vi "Get Device ID.vi"(8 "Error In":errorcluster, 11 "LINX Device Config":T1) -> (0 "Error Out":errorcluster, 2 "Device Name":string, 3 "LINX Device Config":T1)   [LabVIEW 2011, in "LVH-LINX.lvlib" / "Device.lvlib"]
uses:
  Device.lvlib
  Type Defs/LINX Device Config.ctl
  Type Defs/Interface.ctl
  Type Defs/TCP Config.ctl
  Type Defs/Device Family.ctl
  Type Defs/Error Type.ctl
  LVH-LINX.lvlib
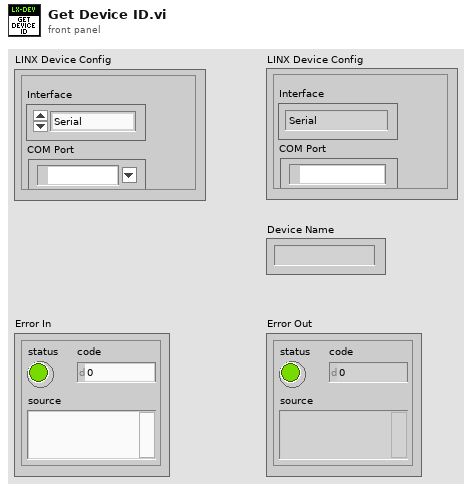
[diagram p1: front panel]
types:
  T1 = typedef "LVH-LINX.lvlib/Device.lvlib/LINX Device Config.ctl" = cluster{"Interface":T2, "COM Port":refnum<visa-resource-name>, "TCP Configuration":T3, "Device Family":T4, "Device ID":u8, "Device Name":string, "TCP Ref":refnum<k5>}
  T2 = typedef "LVH-LINX.lvlib/Interface.ctl" = enum16{"Serial", "TCP"}
  T3 = typedef "LVH-LINX.lvlib/Device.lvlib/TCP Config.ctl" = cluster{"IP Address":string, "Port":u16}
  T4 = typedef "LVH-LINX.lvlib/Device Family.ctl" = enum8{"National Instruments", "Digilent", "Arduino"}
  T5 = typedef "LVH-LINX.lvlib/Error Type.ctl" = enum16{"Unknown", "Timeout", "Corrupt Return Packet", "Unable To Connect", "Command Not Supported", "Channel DNE"}
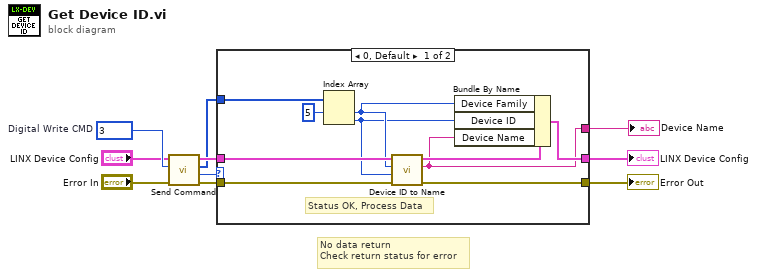
[diagram p0: block diagram]
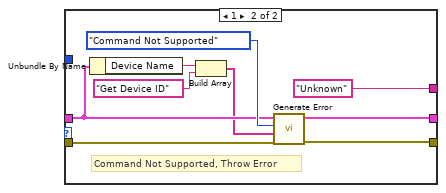
[diagram p2: hidden frame]
diagram:
  w9 = u16 3  # Digital Write CMD
  # "No data return\nCheck return status for error"
  n1 = call "Send Command.vi"("Error In"="Error In", "CMD"=w9, "LINX Device Config"="LINX Device Config") -> ("Error Out"=w4:errorcluster, "Status"=w1:u8, "Response"=w3:u8[], "LINX Device Config"=w6:T1)  [unwired: 5 in]
  n2 = case shown="0, Default" w1 {
    tunnel: [w14 w27] -> w7
    tunnel: w6 -> [w18 w22]
    tunnel: [w16 w28] -> w5
    tunnel: w4 -> [w17 w29]
    tunnel: w3 -> [w20 _]
    tunnel: [w11 "Unknown" ("Device Name")] -> w2
    frame 0, Default {
      # "Status OK, Process Data"
      n3 = Index Array(array=w20, index #1=5 ("index")) -> (element #1=w13:u8, element #2=w12:u8)  [unwired: 1 in]
      n4 = call "Device ID to Name.vi"("Error In"=w17, "Device ID"=w12, "Device Family"=w13, "LINX Device Config"=w18) -> ("Error Out"=w16:errorcluster, "Device Name"=w11:string, "LINX Device Config"=w15:T1)  [unwired: 4 in, 1 out]
      n5 = Bundle By Name(cluster=w15, "Device Family"=w13, "Device ID"=w12, "Device Name"=w11) -> (w14:T1)
    }
    frame 1 {
      # "Command Not Supported, Throw Error"
      n6 = Unbundle By Name(w22) -> ("Device Name"=w23:string)
      n7 = Build Array(w23, "Get Device ID") -> (w21:string[])
      n8 = call "Generate Error.vi"("Error In"=w29, "Arguments"=w21, "Error Type"=Error_Type."Command Not Supported", "LINX Device Config"=w22) -> ("Error Out"=w28:errorcluster, "LINX Device Config"=w27:T1)  [unwired: 6 in]
    }
  }
  "Error Out" <- w5
  "LINX Device Config" <- w7
  "Device Name" <- w2
